vi "main.vi"() -> ()   [LabVIEW 2021]
uses:
  ConfigVISA.ctl
  ConfigNI.ctl
  DAQ_class/DAQ.lvclass
  <vilib>/Analysis/baseanly.llb/Mean (DBL).vi
  <vilib>/Analysis/NI_AALBase.lvlib
panel:
  out "Waveform Chart 0":dbl(graph)
  out "Waveform Graph 0":dynamicdata(graph)
  out "Waveform Chart 1":dbl(graph)
  out "Waveform Graph 1":dynamicdata(graph)
  in  "ConfigNI":T1={"Physical Channels"="", "Number of Samples"=500, "Desired Sample Rate (Hz)"=5000.0, "Minimum Value"=0.0, "Maximum Value"=10.0, "Input Terminal Configuration"=10083, "Sample Mode"=10123, "DAQmx Task Name"=""} {"Sample Mode" items=["Finite Samples"=10178, "Continuous Samples"=10123, "Hardware Timed Single Point"=12522]; "Input Terminal Configuration" items=["Default"=-1, "RSE"=10083, "NRSE"=10078, "Differential"=10106, "Pseudodifferential"=12529]}
  in  "ConfigVISA":T2={"VISA Resource Name"="", "baud rate"=2400, "data bits"=7, "parity"=2, "stop bits"=10, "flow control"=0, "delay before read (ms) 2"=500, "Write Buffer"="Q\r\n"} {"flow control" items=["None"=0, "XON/XOFF"=1, "RTS/CTS"=2, "DTR/DSR"=4]; "stop bits" items=["1.0"=10, "1.5"=15, "2.0"=20]; "parity" items=["None", "Odd", "Even", "Mark", "Space"]; "data bits" min=5 max=8 step=1}
  out "Scales (g)":dbl(slide) scale=0.0..1000.0
  in  "stop":bool
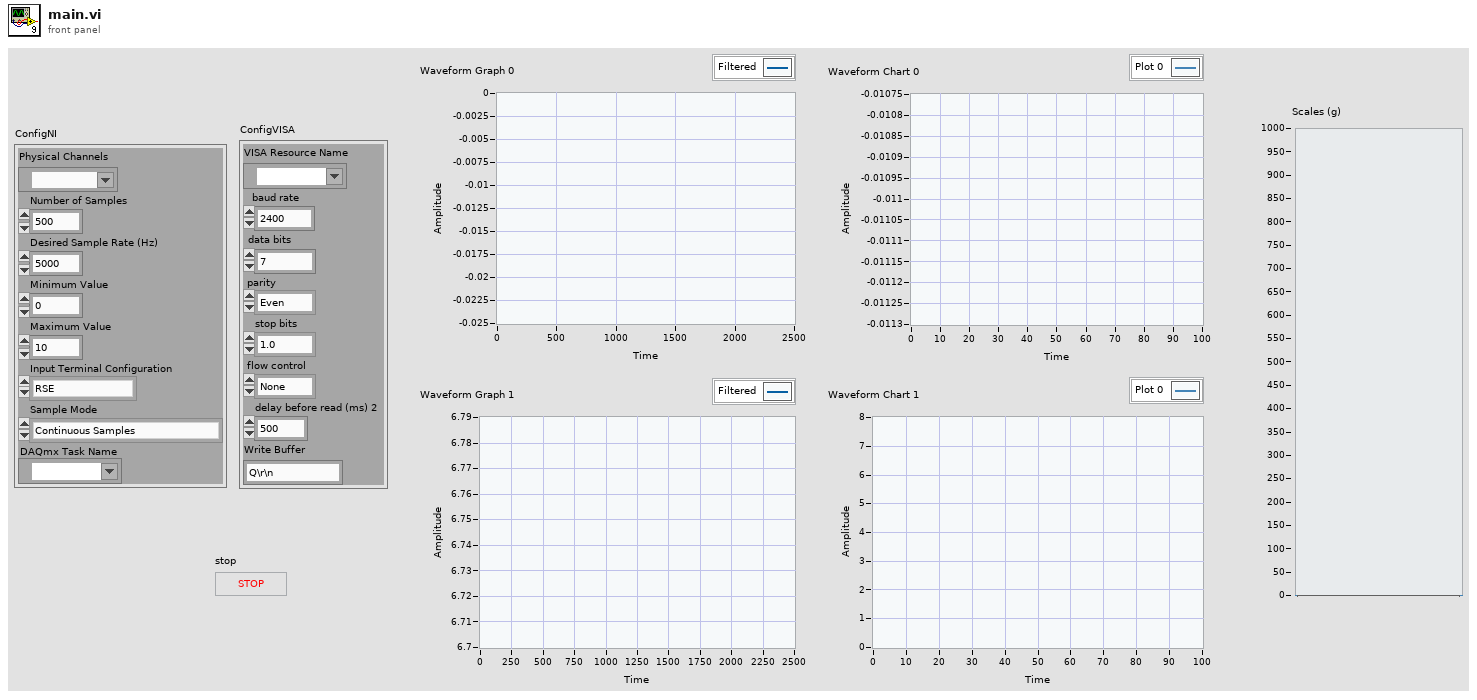
[diagram p1: front panel]
types:
  T1 = typedef "ConfigNI.ctl" = cluster{"Physical Channels":tag, "Number of Samples":i32, "Desired Sample Rate (Hz)":dbl, "Minimum Value":dbl, "Maximum Value":dbl, "Input Terminal Configuration":i32, "Sample Mode":i32, "DAQmx Task Name":refnum<k21>}
  T2 = typedef "ConfigVISA.ctl" = cluster{"VISA Resource Name":refnum<visa-resource-name>, "baud rate":u32, "data bits":u16, "parity":u16, "stop bits":u16, "flow control":u16, "delay before read (ms) 2":u32, "Write Buffer":string}
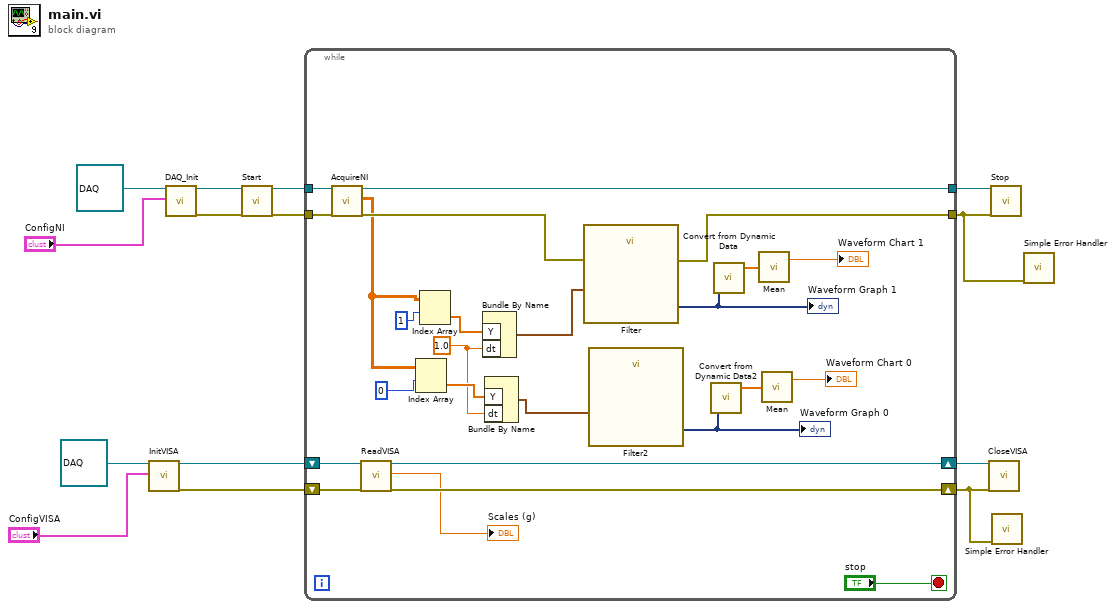
[diagram p0: block diagram]
diagram:
  n1 = call-dynamic "InitVISA.vi"("object in"=refnum<class "DAQ.lvclass"> refnum ("DAQ"), "ConfigVISA"="ConfigVISA") -> ("object out"=w12:refnum<class "DAQ.lvclass">, "error out"=w4:errorcluster)  [unwired: 16 in]
  n2 = call "DAQ_Init.vi"("object in"=refnum<class "DAQ.lvclass"> refnum ("DAQ"), "ConfigNI"="ConfigNI") -> ("object out"=w8:refnum<class "DAQ.lvclass">, "error out"=w7:errorcluster)  [unwired: 16 in]
  n3 = call-dynamic "Start.vi"("object in"=w8, "error in (no error)"=w7) -> ("object out"=w6:refnum<class "DAQ.lvclass">, "error out"=w5:errorcluster)  [unwired: 16 in]
  n4 = while {
    tunnel: [w29] -> w9
    tunnel: [w32] -> w10
    tunnel: w6 -> [w34]
    tunnel: w5 -> [w33]
    shift-right: [w38] -> w11
    shift-left: w12 -> [w39]
    shift-right: [w36] -> w3
    shift-left: w4 -> [w37]
    stop <- "stop" stop-if-true
    w22 = 1.0 ("dt")
    n5 = call-dynamic "AcquireNI.vi"("object in"=w34, "error in (no error)"=w33) -> ("object out"=w32:refnum<class "DAQ.lvclass">, "data"=w26:dbl[][], "error out"=w30:errorcluster)  [unwired: 15 in]
    n6 = call-dynamic "ReadVISA.vi"("object in"=w39, "error in (no error)"=w37) -> ("object out"=w38:refnum<class "DAQ.lvclass">, "Scale Data"=→"Scales (g)":dbl, "error out"=w36:errorcluster)  [unwired: 15 in]
    n7 = Index Array(array=w26, index (row)=0) -> (element=w23:dbl[])  [unwired: 1 in]
    n8 = Index Array(array=w26, index (row)=1) -> (element=w28:dbl[])  [unwired: 1 in]
    n9 = Bundle By Name("Y"=w28, "dt"=w22) -> (w24:waveform(dbl))  [unwired: 1 in]
    n10 = Bundle By Name("Y"=w23, "dt"=w22) -> (w21:waveform(dbl))  [unwired: 1 in]
    n11 = call "Filter"("error in (no error)"=w30, "Signal"=w24) -> ("error out"=w29:errorcluster, "Filtered Signal"=w20:dynamicdata)  [unwired: 8 in]
    "Waveform Graph 1" <- w20
    n12 = call "Filter2"("Signal"=w21) -> ("Filtered Signal"=w17:dynamicdata)  [unwired: 9 in, 1 out]
    "Waveform Graph 0" <- w17
    n13 = call "Convert from Dynamic Data2"("Dynamic Data Type"=w17) -> ("Array"=w16:dbl[])  [unwired: 3 in]
    n14 = call "Convert from Dynamic Data"("Dynamic Data Type"=w20) -> ("Array"=w19:dbl[])  [unwired: 3 in]
    n15 = call-poly <vilib>:"Mean.vi"("X"=w19) -> ("mean"=→"Waveform Chart 1":dbl)  [unwired: 1 out]
    n16 = call-poly <vilib>:"Mean.vi"("X"=w16) -> ("mean"=→"Waveform Chart 0":dbl)  [unwired: 1 out]
  }
  n17 = call-dynamic "CloseVISA.vi"("object in"=w11, "error in (no error)"=w3) -> ()  [unwired: 16 in, 2 out]
  n18 = call-dynamic "Stop.vi"("object in"=w10, "error in (no error)"=w9) -> ()  [unwired: 16 in, 2 out]
  n19 = call <vilib>:"Simple Error Handler.vi"("error in (no error)"=w3) -> ()  [unwired: 4 in, 5 out]
  n20 = call <vilib>:"Simple Error Handler.vi"("error in (no error)"=w9) -> ()  [unwired: 4 in, 5 out]
